vi "niFpga wdp fft streaming bf core dummy.vi"(4 "index=0?":bool, 6 "enable":bool, 8 "switch":bool[](array[boolean])=[FALSE, FALSE, FALSE, FALSE, FALSE, FALSE, FALSE, FALSE, FALSE, FALSE, FALSE, FALSE, FALSE, FALSE, FALSE], 9 "twiddle factors":T3(array[cluster])=[{"tf re"=0.0, "tf im"=0.0}, {"tf re"=0.0, "tf im"=0.0}, {"tf re"=0.0, "tf im"=0.0}, {"tf re"=0.0, "tf im"=0.0}, {"tf re"=0.0, "tf im"=0.0}, {"tf re"=0.0, "tf im"=0.0}, {"tf re"=0.0, "tf im"=0.0}, {"tf re"=0.0, "tf im"=0.0}, {"tf re"=0.0, "tf im"=0.0}, {"tf re"=0.0, "tf im"=0.0}, {"tf re"=0.0, "tf im"=0.0}, {"tf re"=0.0, "tf im"=0.0}, {"tf re"=0.0, "tf im"=0.0}, {"tf re"=0.0, "tf im"=0.0}], 10 "data in 1":T4, 11 "data in 0":T4) -> (2 "data out 1":T1, 3 "data out 0":T2)   [LabVIEW 2017]
types:
  T1 = cluster{"x-y":fxp<+/-,19,12>, "x-y":fxp<+/-,19,12>}
  T2 = cluster{"x+y":fxp<+/-,19,12>, "x+y":fxp<+/-,19,12>}
  T3 = cluster{"tf re":fxp<+/-,16,2>, "tf im":fxp<+/-,16,2>}[]
  T4 = cluster{"data re":fxp<+/-,8,1>, "data im":fxp<+/-,8,1>}
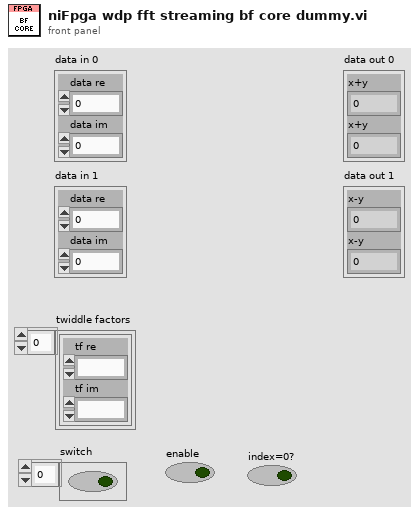
[diagram p1: front panel]
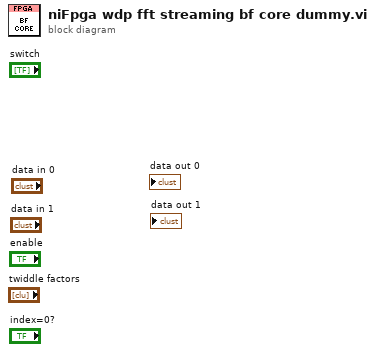
[diagram p0: block diagram]
diagram:
